vi "Load.vi"(8 "error in (no error)":errorcluster, 9 "Channel Name":string, 10 "Group Name":string, 11 "tdms file in":refnum<k34>) -> (0 "error out":errorcluster, 2 "Channel out":refnum<class "Channel.lvclass">, 3 "tdms file out":refnum<k34>)   [LabVIEW 2020, in "TDMS.lvlib" / "Channel.lvclass"]
doc: "Load 'Channel out' data from 'TDMS file in'."
uses:
  Channel.lvclass
  PPL/HDH.Data.Generic.lvlibp/Generic Data/Generic Array Data/Generic Array Data.lvclass
  Channel.lvclass/Channel.ctl
  PPL/HDH.Data.Generic.lvlibp/Generic Data/Generic Array Data/I32 Array/I32 Array.lvclass
  C:/Current projects/WS/PPL/HDH.Data.Generic.lvlibp/Generic Data/Generic Array Data/Generic Array Data.lvclass
  PPL/HDH.Data.Generic.lvlibp/Generic Data/Generic Array Data/Double Array/Double Array.lvclass
  PPL/HDH.Data.Generic.lvlibp/Generic Data/Generic Array Data/Boolean Array/Boolean Array.lvclass
  PPL/HDH.Data.Generic.lvlibp/Generic Data/Generic Array Data/U32 Array/U32 Array.lvclass
  PPL/HDH.Data.Generic.lvlibp/Generic Data/Generic Array Data/String Array/String Array.lvclass
  PPL/HDH.Data.Generic.lvlibp/Generic Data/Generic Array Data/Time Stamp Array/Time Stamp Array.lvclass
  PPL/HDH.Data.Generic.lvlibp/Utility/Wrap In Generic.vi
  PPL/HDH.Data.Generic.lvlibp/Generic Data/Variant/Set Attribute.vi
  PPL/HDH.Data.Generic.lvlibp/Generic Data/Variant/Variant.lvclass
  TDMS.lvlib
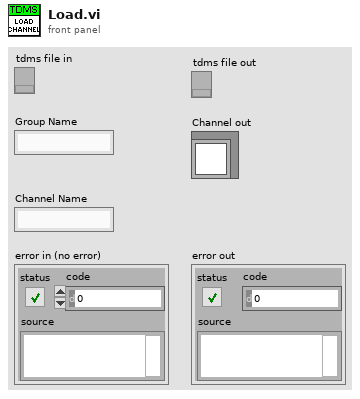
[diagram p1: front panel]
types:
  T1 = typedef "TDMS.lvlib/Ctl_DataType.ctl" = enum16{"void", "int8", "int16", "int32", "int64", "uint8", "uint16", "uint32", "uint64", "single", "double", "extended float", "single with unit", "double with unit", "extended float with unit", "string", "logical", "timestamp", "DAQmx"}
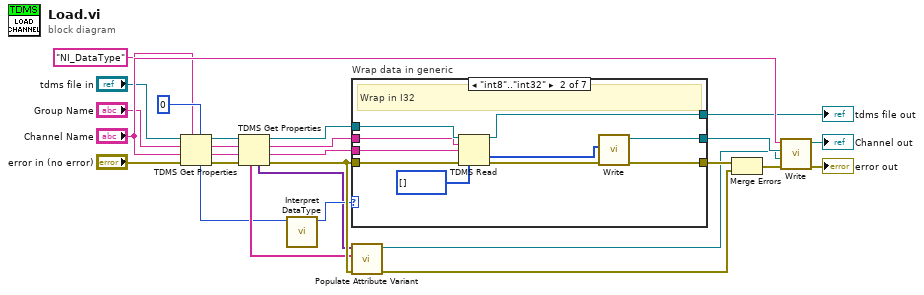
[diagram p0: block diagram]
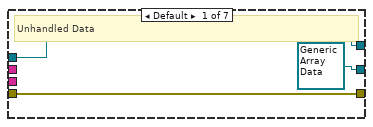
[diagram p2: hidden frame]
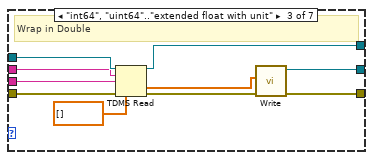
[diagram p3: hidden frame]
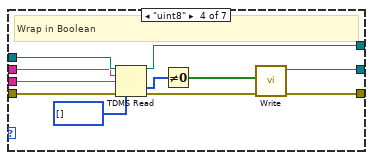
[diagram p4: hidden frame]
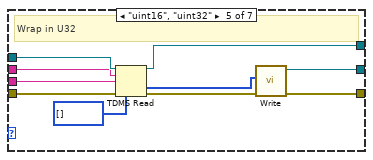
[diagram p5: hidden frame]
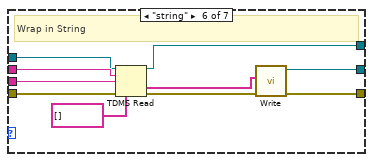
[diagram p6: hidden frame]
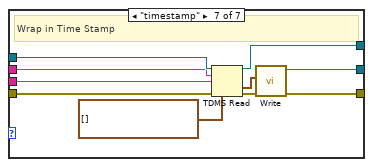
[diagram p7: hidden frame]
diagram:
  n1 = TDMS Get Properties(5:u16 0, 7:"NI_DataType" ("property name"), 8:"error in (no error)", 9:"Channel Name", 10:"Group Name", 11:"tdms file in") -> (0:w7:errorcluster, 1:w9:string, 2:w8:string, 3:w6:refnum<k34>, 4:w5:u16)  [unwired: 1 out]
  n2 = TDMS Get Properties(8:w7, 9:w9, 10:w8, 11:w6) -> (0:w18:errorcluster, 1:w16:string, 2:w15:string, 3:w14:refnum<k34>, 4:w10:variant[], 6:w11:string[])  [unwired: 2 in]
  n3 = call "Interpret DataType.vi"("NI_DataType"=w5) -> ("TDMS Data Type"=w13:T1)  [unwired: 10 in]
  n4 = case "Wrap data in generic" shown="\"int8\"..\"int32\"" w13 {
    tunnel: w14 -> [w27 w38 w45 w57 w65 w71 w84]
    tunnel: w15 -> [_ w31 w44 w56 w63 w72 w83]
    tunnel: w16 -> [_ w32 w43 w55 w62 w73 w82]
    tunnel: [refnum<class "Generic Array Data.lvclass"> refnum ("HDH.Data.Generic.lvlibp:Generic Array Data.lvclass") w36 w40 w49 w59 w68 w77] -> w17
    tunnel: w18 -> [w28 w33 w46 w54 w61 w74 w81]
    tunnel: [w27 w37 w42 w52 w64 w70 w79] -> w19
    tunnel: [w28 w30 w39 w48 w58 w67 w76] -> w21
    frame Default {
      # "Unhandled Data"
    }
    frame "int8".."int32" {
      # "Wrap in I32"
      n5 = TDMS Read(0:w38, 5:w31, 7:w32, 11:w33, 12:i32[] []) -> (4:w37:refnum<k34>, 10:w34:i32[], 15:w30:errorcluster)  [unwired: 3 in, 3 out]
      n6 = call "Write.vi"("I32 Array"=w34) -> ("I32 Array out"=w36:refnum<class "I32 Array.lvclass">)  [unwired: 10 in]
    }
    frame "int64", "uint64".."extended float with unit" {
      # "Wrap in Double"
      n7 = TDMS Read(0:w45, 5:w44, 7:w43, 11:w46, 12:dbl[] []) -> (4:w42:refnum<k34>, 10:w41:dbl[], 15:w39:errorcluster)  [unwired: 3 in, 3 out]
      n8 = call "Write.vi"("Double Array"=w41) -> ("Double Array out"=w40:refnum<class "Double Array.lvclass">)  [unwired: 10 in]
    }
    frame "uint8" {
      # "Wrap in Boolean"
      n9 = TDMS Read(0:w57, 5:w56, 7:w55, 11:w54, 12:u8[] []) -> (4:w52:refnum<k34>, 10:w51:u8[], 15:w48:errorcluster)  [unwired: 3 in, 3 out]
      n10 = Not Equal To 0?(x=w51) -> (x != 0?=w50:bool[])
      n11 = call "Write.vi"("Boolean Array"=w50) -> ("Boolean Array out"=w49:refnum<class "Boolean Array.lvclass">)  [unwired: 10 in]
    }
    frame "uint16", "uint32" {
      # "Wrap in U32"
      n12 = TDMS Read(0:w65, 5:w63, 7:w62, 11:w61, 12:u32[] []) -> (4:w64:refnum<k34>, 10:w60:u32[], 15:w58:errorcluster)  [unwired: 3 in, 3 out]
      n13 = call "Write.vi"("U32 Array"=w60) -> ("U32 Array out"=w59:refnum<class "U32 Array.lvclass">)  [unwired: 10 in]
    }
    frame "string" {
      # "Wrap in String"
      n14 = TDMS Read(0:w71, 5:w72, 7:w73, 11:w74, 12:string[] []) -> (4:w70:refnum<k34>, 10:w69:string[], 15:w67:errorcluster)  [unwired: 3 in, 3 out]
      n15 = call "Write.vi"("String Array"=w69) -> ("String Array out"=w68:refnum<class "String Array.lvclass">)  [unwired: 10 in]
    }
    frame "timestamp" {
      # "Wrap in Time Stamp"
      n16 = TDMS Read(0:w84, 5:w83, 7:w82, 11:w81, 12:timestamp[] []) -> (4:w79:refnum<k34>, 10:w78:timestamp[], 15:w76:errorcluster)  [unwired: 3 in, 3 out]
      n17 = call "Write.vi"("String Array"=w78) -> ("String Array out"=w77:refnum<class "Time Stamp Array.lvclass">)  [unwired: 10 in]
    }
  }
  "tdms file out" <- w19
  n18 = call "Populate Attribute Variant.vi"("error in (no error)"=w18, "Property Names"=w11, "Property Values"=w10) -> ("error out"=w20:errorcluster, "Attribute Variant out"=w12:refnum<class "Variant.lvclass">)  [unwired: 7 in]
  n19 = Merge Errors(w21, w20) -> (w22:errorcluster)
  n20 = call "Write.vi"("error in (no error)"=w22, "Channel Properties"=w12, "Array Data"=w17, "Channel Name"="Channel Name") -> ("error out"=→"error out":errorcluster, "TDMS Channel out"=→"Channel out":refnum<class "Channel.lvclass">)  [unwired: 6 in]
